vi "VerifInstrErrors.vi"(8 "error in (no error)":errorcluster, 11 "S4GUI in":refnum<class "S4GUI.lvclass">) -> (0 "error out":errorcluster, 3 "S4GUI out":refnum<class "S4GUI.lvclass">)   [LabVIEW 2018, in "S4GUI.lvclass"]
uses:
  S4GUI.lvclass
  S4GUI.lvclass/S4GUI.ctl
  Instrument/Instrument.lvclass/Instrument.ctl
  Device/Optics/Opt_Selector/Opt_Selector.lvclass
  StateMachine/State Machine.lvclass
  Instrument/Instrument.lvclass
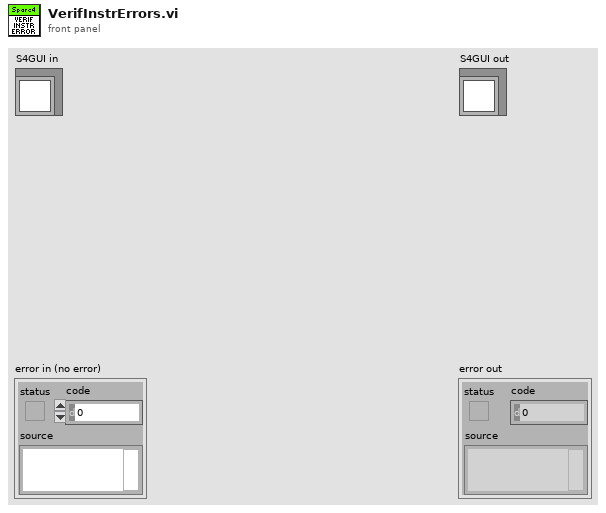
[diagram p1: front panel]
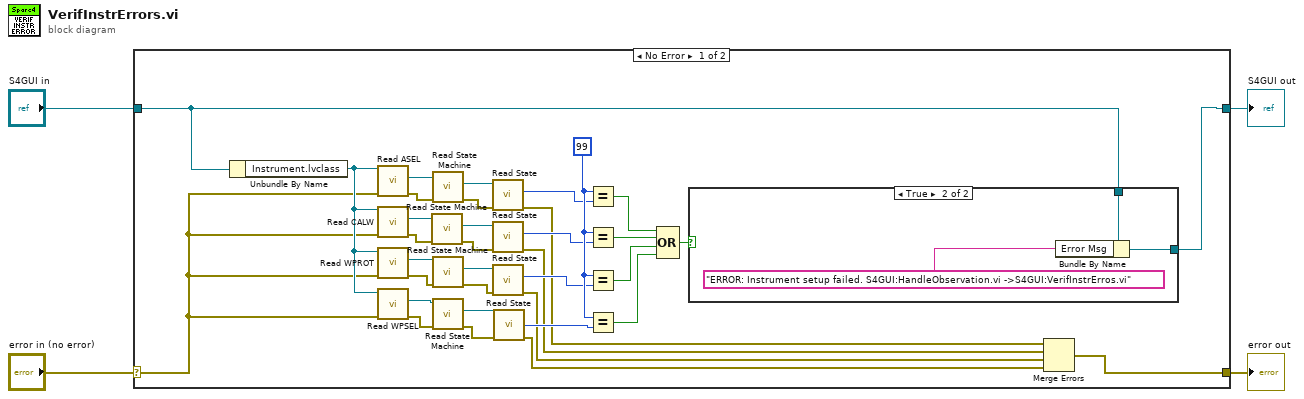
[diagram p0: block diagram]
diagram:
  n1 = case shown="No Error" "error in (no error)" {
    selector: "error in (no error)" -> [w38 w45]
    tunnel: [w37 w45] -> w3
    tunnel: [w9 w44] -> w1
    tunnel: "S4GUI in" -> [w10 w44]
    frame No Error {
      w20 = 99
      n2 = Unbundle By Name(w10) -> ("Instrument.lvclass"=w39:refnum<class "Instrument.lvclass">)
      n3 = call "Read ASEL.vi"("error in (no error)"=w38, "Instrument in"=w39) -> ("error out"=w36:errorcluster, "Opt_Selector.lvclass"=w34:refnum<class "Opt_Selector.lvclass">)  [unwired: 7 in, 1 out]
      n4 = call "Read CALW.vi"("error in (no error)"=w38, "Instrument in"=w39) -> ("error out"=w35:errorcluster, "Opt_Selector.lvclass"=w33:refnum<class "Opt_Selector.lvclass">)  [unwired: 7 in, 1 out]
      n5 = call "Read WPROT.vi"("error in (no error)"=w38, "Instrument in"=w39) -> ("error out"=w31:errorcluster, "Opt_Selector.lvclass"=w32:refnum<class "Opt_Selector.lvclass">)  [unwired: 7 in, 1 out]
      n6 = call "Read WPSEL.vi"("error in (no error)"=w38, "Instrument in"=w39) -> ("error out"=w29:errorcluster, "Opt_Selector.lvclass"=w30:refnum<class "Opt_Selector.lvclass">)  [unwired: 7 in, 1 out]
      n7 = call-dynamic "Read State Machine.vi"("error in (no error)"=w35, "Device in"=w33) -> ("error out"=w25:errorcluster, "State Machine.lvclass"=w26:refnum<class "State Machine.lvclass">)  [unwired: 7 in, 1 out]
      n8 = call-dynamic "Read State Machine.vi"("error in (no error)"=w36, "Device in"=w34) -> ("error out"=w27:errorcluster, "State Machine.lvclass"=w28:refnum<class "State Machine.lvclass">)  [unwired: 7 in, 1 out]
      n9 = call-dynamic "Read State Machine.vi"("error in (no error)"=w31, "Device in"=w32) -> ("error out"=w23:errorcluster, "State Machine.lvclass"=w24:refnum<class "State Machine.lvclass">)  [unwired: 7 in, 1 out]
      n10 = call-dynamic "Read State Machine.vi"("error in (no error)"=w29, "Device in"=w30) -> ("error out"=w21:errorcluster, "State Machine.lvclass"=w22:refnum<class "State Machine.lvclass">)  [unwired: 7 in, 1 out]
      n11 = call-dynamic "Read State.vi"("error in (no error)"=w27, "State Machine in"=w28) -> ("error out"=w8:errorcluster, "State"=w19:i32)  [unwired: 7 in, 1 out]
      n12 = call-dynamic "Read State.vi"("error in (no error)"=w25, "State Machine in"=w26) -> ("error out"=w7:errorcluster, "State"=w18:i32)  [unwired: 7 in, 1 out]
      n13 = call-dynamic "Read State.vi"("error in (no error)"=w23, "State Machine in"=w24) -> ("error out"=w6:errorcluster, "State"=w17:i32)  [unwired: 7 in, 1 out]
      n14 = call-dynamic "Read State.vi"("error in (no error)"=w21, "State Machine in"=w22) -> ("error out"=w5:errorcluster, "State"=w16:i32)  [unwired: 7 in, 1 out]
      n15 = Equal?(x=w20, y=w19) -> (x = y?=w15:bool)
      n16 = Equal?(x=w20, y=w18) -> (x = y?=w14:bool)
      n17 = Equal?(x=w20, y=w17) -> (x = y?=w13:bool)
      n18 = Equal?(x=w20, y=w16) -> (x = y?=w12:bool)
      n19 = Compound Arithmetic op=OR(w15, w14, w13, w12) -> (w11:bool)
      n20 = case shown="True" w11 {
        tunnel: w10 -> [w40 w43]
        tunnel: [w40 w42] -> w9
        frame False {
        }
        frame True {
          n21 = Bundle By Name(cluster=w43, "Error Msg"="ERROR: Instrument setup failed. S4GUI:HandleObservation.vi ->S4GUI:VerifInstrErros.vi") -> (w42:refnum<class "S4GUI.lvclass">)
        }
      }
      n22 = Merge Errors(w8, w7, w6, w5) -> (w37:errorcluster)
    }
    frame Error {
    }
  }
  "error out" <- w3
  "S4GUI out" <- w1
